vi "Do.vi"(8 "error in (no error)":errorcluster, 10 "Actor in":refnum<class "Actor.lvclass">, 11 "MainPane Slide Msg":refnum<class "MainPane Slide Msg.lvclass">) -> (0 "error out":errorcluster, 2 "Actor out":refnum<class "Actor.lvclass">)   [LabVIEW 2012, in "Win8uiFramework.lvlib" / "MainPane Slide Msg.lvclass"]
doc: "This VI delivers the message to the actor by calling the appropriate method(s) on the actor."
uses:
  MainPane Slide Msg.lvclass
  <vilib>/ActorFramework/Actor/Actor.lvclass
  MainController.lvclass
  MainPane Slide Msg.lvclass/MainPane Slide Msg.ctl
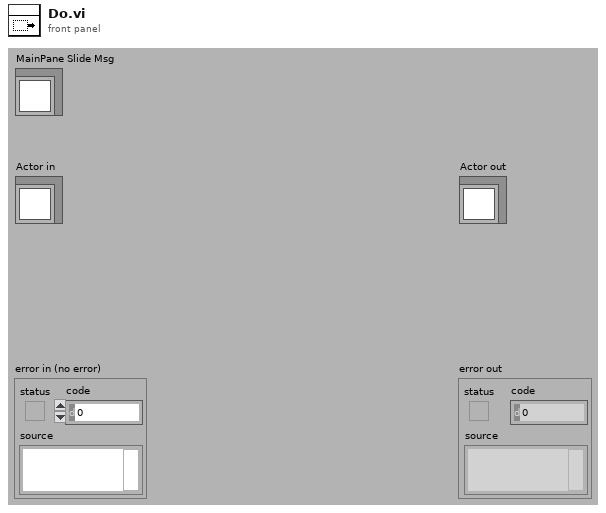
[diagram p1: front panel]
types:
  T1 = typedef "Win8uiFramework.lvlib/Slide Direction.ctl" = enum16{"Forwards", "Back"}
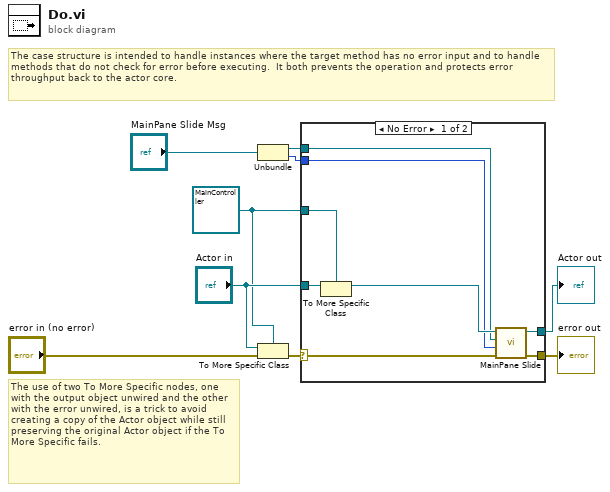
[diagram p0: block diagram]
diagram:
  w4 = refnum<class "MainController.lvclass"> refnum ("Actor in")
  # "The use of two To More Specific nodes, one with the output object unwired and the other with the error unwired, is a trick to avoid creating a copy of the Actor object while still preserving the original Actor object if the To More Specific fails."
  # "The case structure is intended to handle instances where the target method has no error input and to handle methods that do not check for error before executing.  It both prevents the operation and protects error throughput back to the actor core."
  n1 = Unbundle("MainPane Slide Msg") -> (w3:refnum<class "Message Enqueuer.lvclass">, w2:T1)
  n2 = To More Specific Class(target class=w4, reference="Actor in", error in="error in (no error)") -> (error out=w8:errorcluster)  [unwired: 1 out]
  n3 = case shown="No Error" w8 {
    selector: w8 -> [w15 w19]
    tunnel: [w17 w19] -> w7
    tunnel: [w16 w18] -> w6
    tunnel: "Actor in" -> [w14 w18]
    tunnel: w4 -> [w13 _]
    tunnel: w3 -> [w11 _]
    tunnel: w2 -> [w10 _]
    frame No Error {
      n4 = To More Specific Class(target class=w13, reference=w14) -> (specific class reference=w12:refnum<class "MainController.lvclass">)  [unwired: 1 in, 1 out]
      n5 = call-dynamic "MainPane Slide.vi"("error in (no error)"=w15, "Slide Direction"=w10, "Enqueuer"=w11, "MainController in"=w12) -> ("error out"=w17:errorcluster, "MainController out"=w16:refnum<class "MainController.lvclass">)  [unwired: 6 in]
    }
    frame Error {
      # "If type check fails, pass the original object out again."
    }
  }
  "error out" <- w7
  "Actor out" <- w6
